vi "webcam_acquire_image.vi"(8 "Image name":string, 11 "store path":path) -> (2 "Image full path":path, 3 "Image Out":T1)   [LabVIEW 2017]
uses:
  <vilib>/vision/Image Controls.llb/IMAQ Image.ctl
panel:
  out "error out":errorcluster
  out "Image":T1(plugin-control)
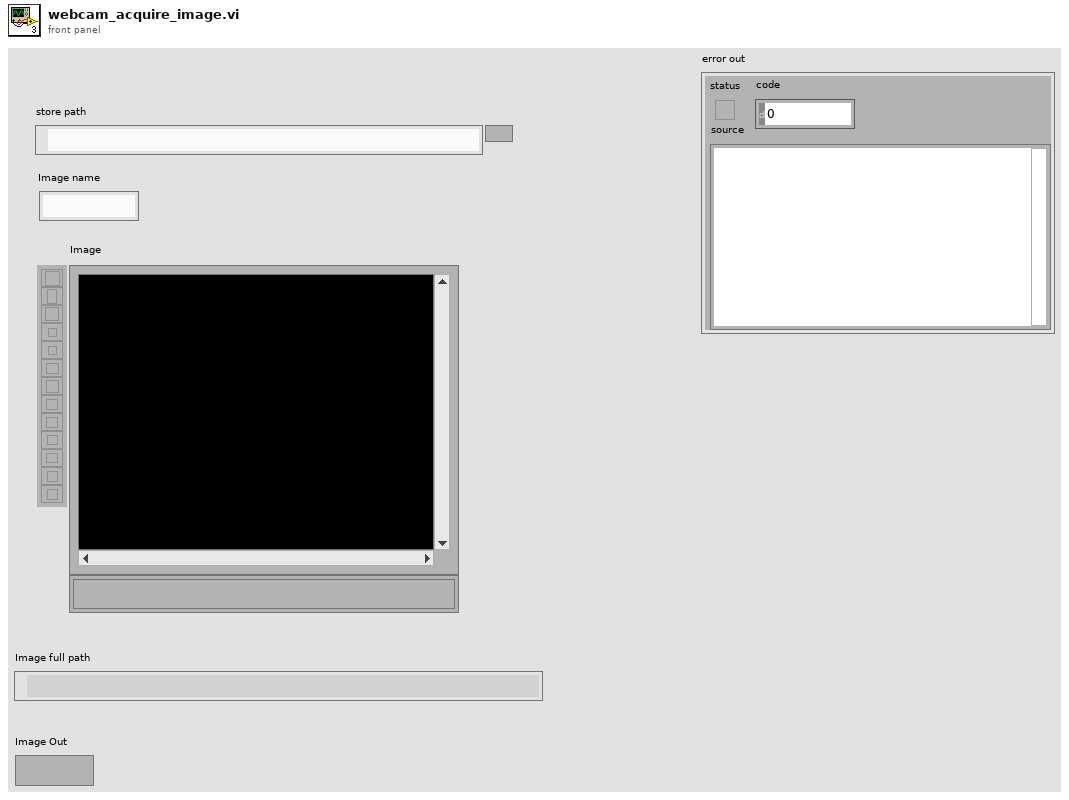
[diagram p1: front panel]
types:
  T1 = typedef "IMAQ Image.ctl" = refnum<image>
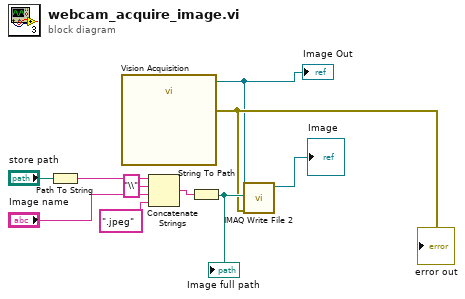
[diagram p0: block diagram]
diagram:
  n1 = Path To String(path="store path") -> (string=w5:string)
  n2 = call "Vision Acquisition"() -> ("Image Out"=w2:T1, "error out"=w3:errorcluster)  [unwired: 26 in]
  "Image Out" <- w2
  "error out" <- w3
  n3 = Concatenate Strings(w5, "\\" ("string"), "Image name", ".jpeg" ("string")) -> (w10:string)
  n4 = String To Path(string=w10) -> (path=w8:path)
  "Image full path" <- w8
  n5 = call-poly "IMAQ Write File 2"("error in (no error)"=w3, "File Path"=w8, "Image"=w2) -> ("Image Out (duplicate)"=→"Image":T1)  [unwired: 7 in, 1 out]
